vi "prueba_dac.vi"() -> ()   [LabVIEW 2025]
panel:
  in  "DAC":u8(knob) scale=0.0..255.0
  in  "stop":bool
  out "Voltaje":dbl
  in  "Pin":u8=25 min=25 max=26
  in  "VISA resource name":refnum<visa-resource-name>
  out "error out":errorcluster
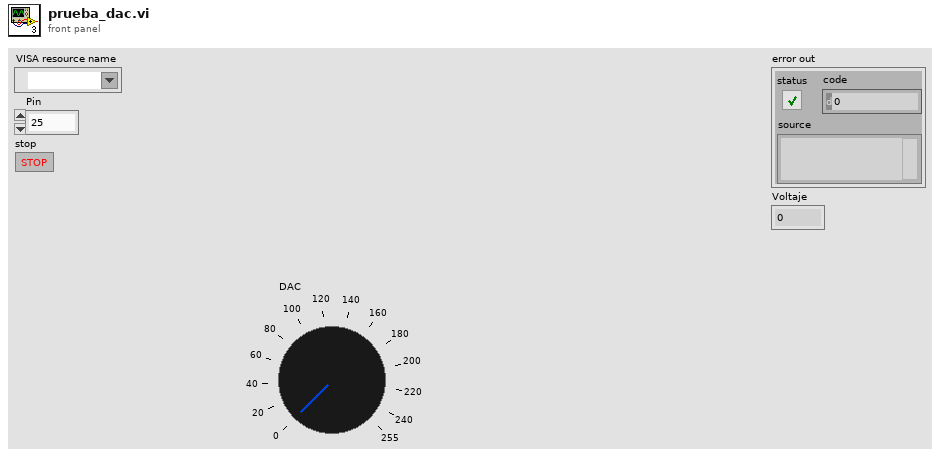
[diagram p1: front panel]
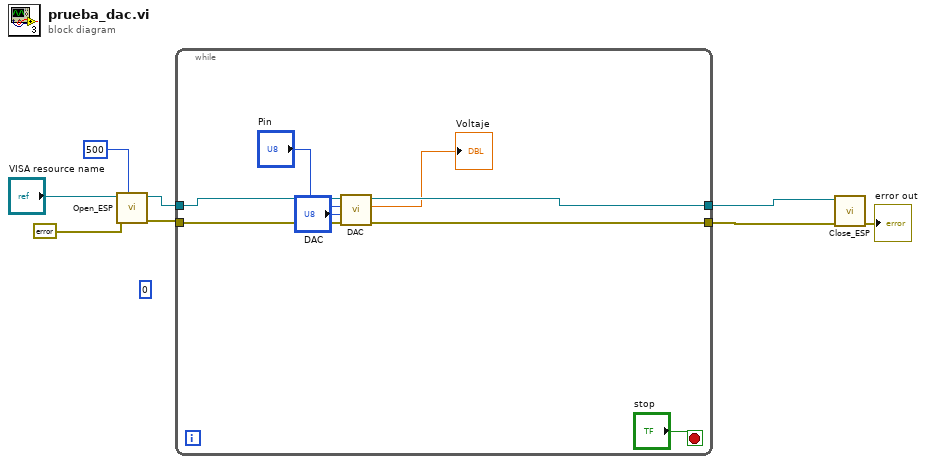
[diagram p0: block diagram]
diagram:
  (unwired) u32 0 ("timeout (10sec)")
  n1 = call "Open_ESP.vi"("timeout (10sec)"=u32 500, "error in (no error)"=errorcluster {"status"=FALSE, "code"=0, "source"=""}, "VISA resource name"="VISA resource name") -> ("error out"=w7:errorcluster, "VISA resource name out"=w8:refnum<visa-resource-name>)  [unwired: 7 in]
  n2 = while {
    tunnel: w8 -> [w16]
    tunnel: [w14] -> w6
    tunnel: w7 -> [w15]
    tunnel: [w13] -> w5
    stop <- "stop" stop-if-true
    n3 = call "DAC.vi"("error in (no error)"=w15, "DAC"="DAC", "Pin"="Pin", "VISA resource name"=w16) -> ("error out"=w13:errorcluster, "Voltaje"=→"Voltaje":dbl, "VISA resource name out"=w14:refnum<visa-resource-name>)  [unwired: 5 in]
  }
  n4 = call "Close_ESP.vi"("error in (no error)"=w5, "VISA resource name"=w6) -> ("error out"=→"error out":errorcluster)  [unwired: 9 in]
